vi "Nanosleep Relative (seconds).vi"(8 "error in (no error)":errorcluster, 10 "clock id (realtime)":T1, 11 "sleep for (seconds)":dbl=1.0 format="%#_6f") -> (0 "error out":errorcluster)   [LabVIEW 2013, in "Linux RT Utilities.lvlib"]
doc: "This VI sleeps the calling thread for the specified relative time."
uses:
  Linux RT Utilities.lvlib
  Controls/Public/C Enums/clockid_t.ctl
  Controls/Public/nanosleep flags.ctl
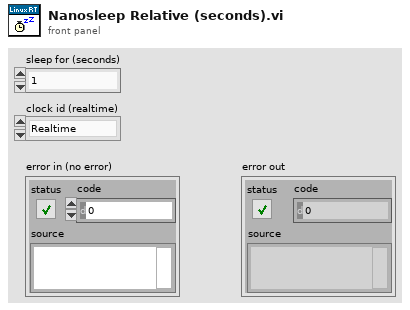
[diagram p1: front panel]
types:
  T1 = typedef "Linux RT Utilities.lvlib/clockid_t.ctl" = enum16{"Realtime", "Monotonic"}
  T2 = typedef "Linux RT Utilities.lvlib/nanosleep flags.ctl" = enum16{"Relative Time", "Absolute Time"}
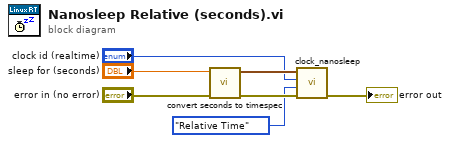
[diagram p0: block diagram]
diagram:
  n1 = call "convert seconds to timespec.vi"("seconds"="sleep for (seconds)") -> ("timespec"=w4:cluster{"sec":u64, "nsec":u64})  [unwired: 10 in]
  n2 = call "clock_nanosleep.vi"("error in (no error)"="error in (no error)", "flags"=nanosleep_flags."Relative Time", "clockid_t"="clock id (realtime)", "request"=w4) -> ("error out"=→"error out":errorcluster)  [unwired: 6 in, 1 out]
